vi "LEBITplc.TrendMessage.vi"(0 "i ref in":refnum<vi>, 1 "data":dbl, 2 "i attribute":T1, 3 "index":i32, 5 "error in":errorcluster, 6 "quality":i32, 9 "no link":bool) -> (14 "i ref out":refnum<vi>, 15 "data out":dbl, 16 "i attribute out":T1, 19 "error out":errorcluster)   [LabVIEW 2014, in "LEBITplc.lvlib"]
uses:
  LEBITplc.lvlib
  LEBITplc.i attribute.ctl
  CSlibraries/UtilityLib/UtilityLib.valueStatus.ctl
  CSlibraries-extern/DimLVEvent/LVDimInterface/LVDimInterface.lvlib
  CSlibraries/UtilityLib/UtilityLib.lvlib
  CSCore/CSSystem/CoreLib/CoreLib.lvlib
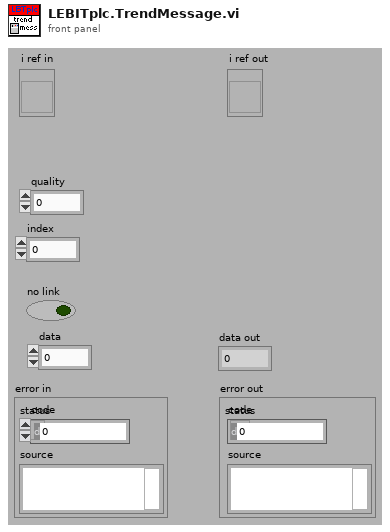
[diagram p1: front panel]
types:
  T1 = typedef "LEBITplc.lvlib/LEBITplc.i attribute.ctl" = cluster{"LLFLocation":string, "SetFileLocation":string, "nickNames":string[], "setValuePLCServiceID":i32[], "GUIServiceID":i32[], "monValuePLC":string[], "SetValueServiceID":i32[], "MonValueServiceID":i32[], "SetValue":dbl[][], "SetValueMin":dbl[], "SetValueMax":dbl[], "SetValueInfoServiceID":i32[], "GUINames":string[], "ListOfBases":string[], "Scale":dbl[], "Offset":dbl[], "setValuePLC":string[], "BaseName":string[], "ScaleServiceID":i32[], "OffsetServiceID":i32[], "AllPLCValues":string[], "CondSpecialArray":string[][], "CondSpecialIndex":i32[], "CondSpecialMonValue":dbl[], "RecentlyChanged":i32[], "SetFileLocationID":i32, "Dependent-Monitors":string[][], "LastLoadedFiles":string[], "IonGuideCalibLocation":string, "Monitor Dependent":string[], "Special":string[], "PLC?":bool[], "Start Date":string, "ListOfBasesServiceID":i32, "SETRA VISA resource":refnum<visa-resource-name>}
  T2 = typedef "UtilityLib.lvlib/UtilityLib.valueStatus.ctl" = enum16{"no info available", "stand by/off", "on", "warning", "alarm/malfunction", "not implemented", "user action required", "important information", "system default", "control default", "indicator default", "button default"}
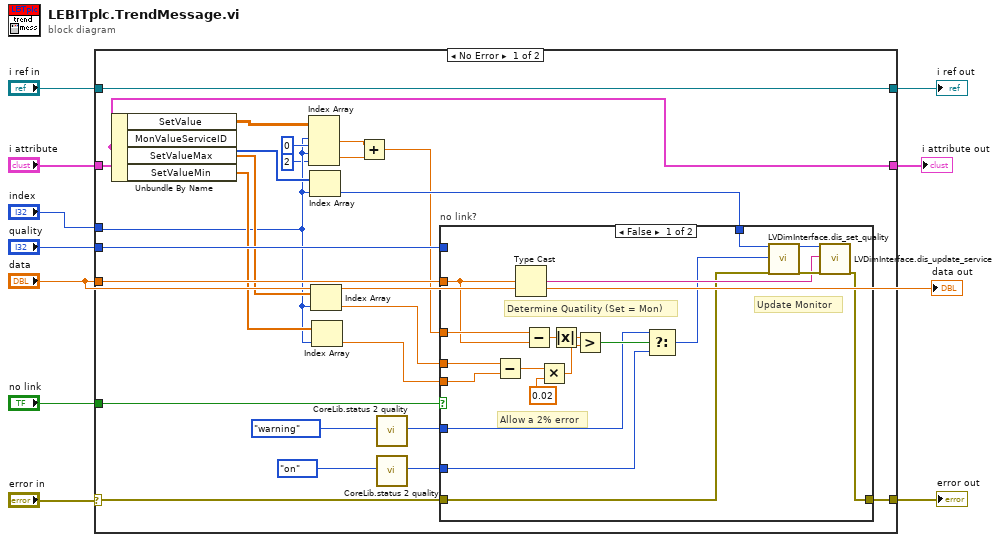
[diagram p0: block diagram]
diagram:
  n1 = case shown="No Error" "error in" {
    selector: "error in" -> [w18 w57]
    tunnel: "quality" -> [w32 _]
    tunnel: "no link" -> [w31 _]
    tunnel: [w19 w57] -> w8
    tunnel: "data" -> [w30 _]
    tunnel: "i attribute" -> [w16 w55]
    tunnel: "i ref in" -> [w17 w56]
    tunnel: [w17 w56] -> w4
    tunnel: "index" -> [w15 _]
    tunnel: [w16 w55] -> w2
    frame No Error {
      n2 = Unbundle By Name(w16) -> ("SetValue"=w33:dbl[][], "MonValueServiceID"=w29:i32[], "SetValueMax"=w28:dbl[], "SetValueMin"=w27:dbl[])
      n3 = Index Array(array=w33, index (row) #1=w15, index (col) #1=0 ("disabled index (col)"), index (row) #2=w15, index (col) #2=2 ("disabled index (col)")) -> (element #1=w13:dbl, element #2=w12:dbl)
      n4 = Index Array(array=w29, index=w15) -> (element=w20:i32)
      n5 = Index Array(array=w28, index=w15) -> (element=w25:dbl)
      n6 = Index Array(array=w27, index=w15) -> (element=w26:dbl)
      n7 = Add(x=w13, y=w12) -> (x+y=w11:dbl)
      n8 = call "CoreLib.status 2 quality.vi"("valueStatus"=UtilityLib.valueStatus."warning") -> ("quality"=w23:i32)  [unwired: 18 in]
      n9 = call "CoreLib.status 2 quality.vi"("valueStatus"=UtilityLib.valueStatus."on") -> ("quality"=w22:i32)  [unwired: 18 in]
      n10 = case "no link?" shown="False" w31 {
        tunnel: w30 -> [w52 _]
        tunnel: w32 -> [_ _]
        tunnel: w11 -> [w53 _]
        tunnel: w22 -> [w51 _]
        tunnel: w26 -> [w50 _]
        tunnel: w25 -> [w49 _]
        tunnel: w23 -> [w35 _]
        tunnel: w20 -> [w47 _]
        tunnel: [w44 w54] -> w19
        tunnel: w18 -> [w36 w54]
        frame False {
          # "Allow a 2% error"
          # "Determine Quatility (Set = Mon)"
          # "Update Monitor"
          n11 = Subtract(x=w49, y=w50) -> (x-y=w41:dbl)
          n12 = Type Cast(x=w52) -> (*(type *) &x=w45:string)  [unwired: 1 in]
          n13 = Subtract(x=w53, y=w52) -> (x-y=w43:dbl)
          n14 = Multiply(x=w41, y=0.02) -> (x*y=w39:dbl)
          n15 = Absolute Value(x=w43) -> (abs(x)=w42:dbl)
          n16 = Greater?(x=w42, y=w39) -> (0:w38:bool)
          n17 = Select(t=w35, s=w38, f=w51) -> (s? t:f=w37:i32)
          n18 = call "LVDimInterface.dis_set_quality.vi"("my_serviceID"=w47, "quality"=w37, "error in (no error)"=w36) -> ("my_serviceID (out)"=w46:i32, "error out"=w48:errorcluster)  [unwired: 15 in]
          n19 = call "LVDimInterface.dis_update_service.vi"("my_serviceID"=w46, "data"=w45, "error in (no error)"=w48) -> ("error out"=w44:errorcluster)  [unwired: 14 in, 2 out]
        }
        frame True {
        }
      }
    }
    frame Error {
    }
  }
  "error out" <- w8
  "i ref out" <- w4
  "i attribute out" <- w2
  "data out" <- "data"
